vi "NanotecSMCPD.set axis stop velocity.vi"(0 "i ref in":refnum<vi>, 1 "axis":i32, 2 "velocity [units/s]":dbl=1.0, 3 "ms timeout (10000)":i32=10000, 5 "error in (no error)":errorcluster) -> (14 "i ref out":refnum<vi>, 17 "timed out":bool, 19 "error out":errorcluster)   [LabVIEW 2014, in "NanotecSMCPD.lvlib"]
doc: "For the specified axis, sets the maximum velocity for a trajectory of movement."
uses:
  NanotecSMCPD.lvlib
  CS_Core/CSSystem/CoreDefs/CoreDefs.error_type.ctl
  CS_Core/CSSystem/CoreDefs/CoreDefs.error_severity.ctl
  CS_Core/CSApplicationBaseClasses/MotorBase/MotorBase.directionType.ctl
  CS_Core/CSApplicationBaseClasses/MotorBase/MotorBase.serviceType.ctl
  CS_Core/CSApplicationBaseClasses/DeviceBase/DeviceBase.lvlib
  CS_Core/CSSystem/CoreLib/CoreLib.lvlib
  CS_Core/CSApplicationBaseClasses/MotorBase/MotorBase.lvlib
  instr.lib/NanotecSMCPD/NanotecSMCPDDriver.lvlib
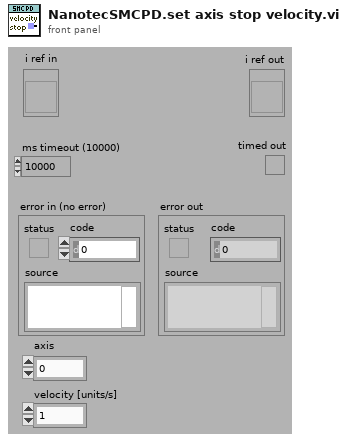
[diagram p1: front panel]
types:
  T1 = typedef "CoreDefs.error_severity.ctl" = enum16{"undefined", "information", "warning", "error", "fatal"}
  T2 = typedef "CoreDefs.error_type.ctl" = enum16{"no error", "can't load process", "can't unload process", "process does not exist", "can't install process", "can't remove process", "unknown function", "time out", "can't execute function", "duplicate queue name", "super not found", "caller queue invalid", "can't ping process", "unknown error", "VISA Error", "VISA timeout", "GPIB timeout", "GPIB error", "communication error", "data type mismatch", "can't read data from OPC server", "can't write data to OPC server", "OET error", "function not implemented", "process already exists", "invalid Shared Variable name", "error writing Shared Variable", "error reading Shared Variable", "invalid client name", "corrupt database", "unknown class", "call not authorized", "parameter out of range", "OET timeout: can't get data to modify", "invalid queue name", "requested operation incompatible with current state", "event undefined", "event disabled", "state undefined", "caller is not a friend", "EventBuilder: bad eventID", "EventBuilder: no DAQ devices", "a thread must not stop itself", "UNUSED ELEMENT4", "DiscArchiver: eventData incomplete", "DiscArchiver: eventData does not belong to run", "DiscArchiver: can't open file", "DiscArchiver: can't write to file", "DiscArchiver: available disc space low", "can't acquire semaphore", "error reading data from database", "notifier object is not existing", "can't register process", "can't unregister process", "illegal event type", "object disabled", "object already exists", "can't change state", "Instrument not found", "no connection to remote node", "invalid reference", "N/A", "UNUSED ELEMENT 1", "element not found", "illegal TCP/IP connection detected", "object does not exist", "invalid access ID", "unknown CS system", "invalid privilige", "unsupported data type", "unsupported server type", "IO server already exists", "Shared Variable already exists"}
  T3 = typedef "MotorBase.lvlib/MotorBase.serviceType.ctl" = enum16{"onOff", "startVelocity", "stopVelocity", "acceleration", "rangeMin", "rangeMax", "status", "position"}
  T4 = typedef "MotorBase.lvlib/MotorBase.directionType.ctl" = enum16{"unknown", "update actual value", "update nominal value", "update both"}
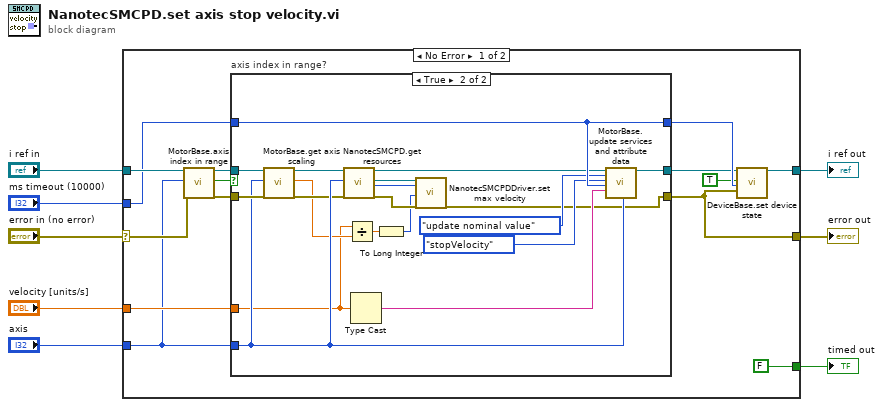
[diagram p0: block diagram]
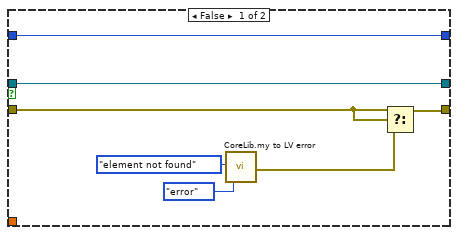
[diagram p2: hidden frame]
diagram:
  n1 = case shown="No Error" "error in (no error)" {
    selector: "error in (no error)" -> [w15 w49]
    tunnel: "ms timeout (10000)" -> [w11 _]
    tunnel: "i ref in" -> [w16 w50]
    tunnel: [w14 w49] -> w5
    tunnel: "axis" -> [w12 _]
    tunnel: [w10 w50] -> w3
    tunnel: "velocity [units/s]" -> [w13 _]
    tunnel: [FALSE ("timed out") _] -> w1
    frame No Error {
      n2 = call "MotorBase.axis index in range.vi"("i ref in"=w16, "axisIndex"=w12, "error in (no error)"=w15) -> ("i ref out"=w20:refnum<vi>, "in range"=w19:bool, "error out"=w21:errorcluster)  [unwired: 14 in]
      n3 = case "axis index in range?" shown="True" w19 {
        tunnel: [w29 w34] -> w18
        tunnel: [w26 w33] -> w14
        tunnel: w11 -> [w23 w48]
        tunnel: w13 -> [_ w35]
        tunnel: w12 -> [_ w39]
        tunnel: w20 -> [w29 w41]
        tunnel: w21 -> [w27 w40]
        tunnel: [w23 w48] -> w22
        frame False {
          n4 = call "CoreLib.my to LV error.vi"("ErrorTypes"=CoreDefs.error_type."element not found", "severityLevel"=CoreDefs.error_severity."error") -> ("myErrorCluster"=w25:errorcluster)  [unwired: 16 in, 1 out]
          n5 = Select(t=w27, s=w27, f=w25) -> (s? t:f=w26:errorcluster)
        }
        frame True {
          n6 = call "MotorBase.get axis scaling.vi"("i ref in"=w41, "axisIndex"=w39, "error in (no error)"=w40) -> ("i ref out"=w38:refnum<vi>, "scaling"=w36:dbl, "error out"=w37:errorcluster)  [unwired: 14 in]
          n7 = call "NanotecSMCPD.get resources.vi"("i ref in"=w38, "axisNumber"=w39, "error in (no error)"=w37) -> ("i ref out"=w42:refnum<vi>, "VISA resource"=w44:refnum<visa-resource-name>, "address"=w32:i32, "error out"=w43:errorcluster)  [unwired: 13 in]
          n8 = Divide(x=w35, y=w36) -> (x/y=w31:dbl)
          n9 = Type Cast(x=w35) -> (*(type *) &x=w47:string)  [unwired: 1 in]
          n10 = To Long Integer(number=w31) -> (32bit integer=w30:i32)
          n11 = call "NanotecSMCPDDriver.set max velocity.vi"("VISA resource name"=w44, "contollerID"=w32, "maxVelocity [Hz]"=w30, "error in (no error)"=w43) -> ("error out"=w33:errorcluster)  [unwired: 13 in, 2 out]
          n12 = call "MotorBase.update services and attribute data.vi"("i ref in"=w42, "direction"=MotorBase.directionType."update nominal value", "service"=MotorBase.serviceType."stopVelocity", "ms timeout (10000)"=w48, "value"=w47, "axisNumber"=w39) -> ("i ref out"=w34:refnum<vi>)  [unwired: 11 in, 2 out]
        }
      }
      n13 = call "DeviceBase.set device state.vi"("i ref in"=w18, "implicit"=TRUE, "ms timeout (10000)"=w22, "device error"=w14) -> ("i ref out"=w10:refnum<vi>)  [unwired: 13 in, 2 out]
    }
    frame Error {
    }
  }
  "error out" <- w5
  "i ref out" <- w3
  "timed out" <- w1
